vi "MTMount_getNextSample_GeneralPurposeGlycolWater.vi"(8 "error in (no error)":errorcluster, 11 "General_Purpose_Glycol_Water_Ctl":T1) -> (0 "error out":errorcluster, 2 "function return":i32, 3 "General_Purpose_Glycol_Water_Ctl out":T1)   [LabVIEW 2018, in "SALLV_MTMount.lvlib"]
doc: "int MTMount_shm_getNextSample_General_Purpose_Glycol_WaterLV(MTMount_General_Purpose_Glycol_WaterLV *General_Purpose_Glycol_Water_Ctl );"
uses:
  SALLV_MTMount.lvlib
  DataTypes/General_Purpose_Glycol_Water.ctl
  SALLV_MTMount.so
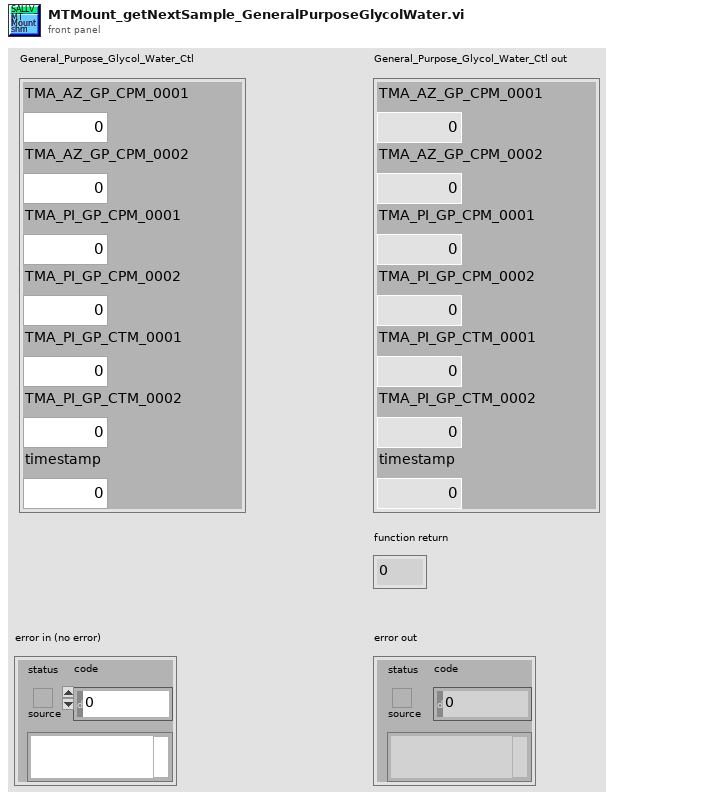
[diagram p1: front panel]
types:
  T1 = typedef "SALLV_MTMount.lvlib/General_Purpose_Glycol_Water.ctl" = cluster{"TMA_AZ_GP_CPM_0001":dbl, "TMA_AZ_GP_CPM_0002":dbl, "TMA_PI_GP_CPM_0001":dbl, "TMA_PI_GP_CPM_0002":dbl, "TMA_PI_GP_CTM_0001":dbl, "TMA_PI_GP_CTM_0002":dbl, "timestamp":dbl}
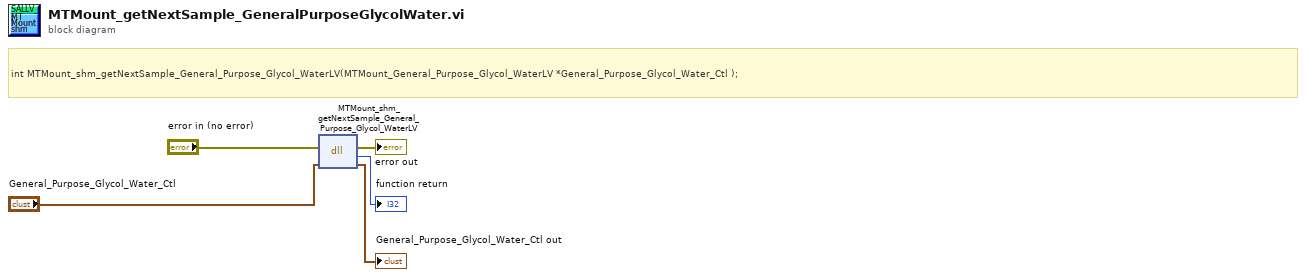
[diagram p0: block diagram]
diagram:
  # "int MTMount_shm_getNextSample_General_Purpose_Glycol_WaterLV(MTMount_General_Purpose_Glycol_WaterLV *General_Purpose_Glycol_Water_Ctl );"
  n1 = dll-call lib="home/ttsai/Document/salApiMTMount/SALLV_MTMount/SALLV_MTMount.*" fn="MTMount_shm_getNextSample_General_Purpose_Glycol_WaterLV"(error in="error in (no error)", "General_Purpose_Glycol_Water_Ctl"="General_Purpose_Glycol_Water_Ctl") -> (error out=→"error out":errorcluster, →"function return":i32, "General_Purpose_Glycol_Water_Ctl"=→"General_Purpose_Glycol_Water_Ctl out":T1)  [unwired: 2 in, 1 out]
